vi "docmd2.vi"(4 "error out 2":errorcluster, 5 "Param":string, 6 "VI_Name":string, 7 "CMDpath":path) -> (1 "rezult":string, 2 "VI Description":string)   [LabVIEW 2010]
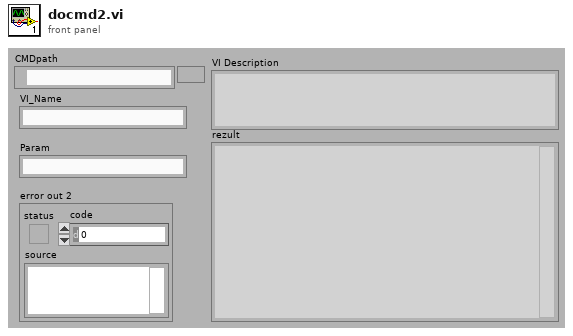
[diagram p1: front panel]
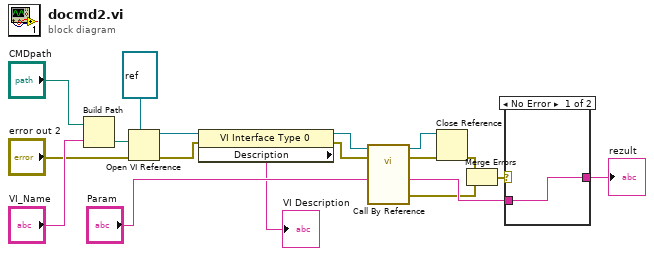
[diagram p0: block diagram]
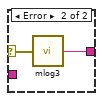
[diagram p2: hidden frame]
diagram:
  n1 = Build Path(base path="CMDpath", name or relative path="VI_Name") -> (appended path=w12:path)
  n2 = Open VI Reference(type specifier VI Refnum (for type only)=refnum<vi> refnum, vi path=w12, error in (no error)="error out 2") -> (vi reference=w6:refnum<vi>, error out=w4:errorcluster)  [unwired: 3 in]
  n3 = property class="VI Interface Type 0"(reference=w6, error in=w4) -> (reference out=w5:refnum<vi>, error out=w3:errorcluster, "Description"=→"VI Description":string)
  n4 = call-by-ref "?"(reference=w5, error in=w3, "Param"="Param") -> (reference out=w8:refnum<vi>, error out=w9:errorcluster, 0:"error out"=w11:errorcluster, "Rezult"=w18:string)  [unwired: 5 in]
  n5 = Close Reference(reference=w8, error in (no error)=w9) -> (error out=w10:errorcluster)
  n6 = Merge Errors(w10, w11) -> (w17:errorcluster)
  n7 = case shown="No Error" w17 {
    selector: w17 -> [_ w21]
    tunnel: w18 -> [w19 _]
    tunnel: [w19 w20] -> w1
    frame No Error {
    }
    frame Error {
      n8 = call "mlog3.vi"("error in"=w21) -> ("message"=w20:string)
    }
  }
  "rezult" <- w1
